vi "MicTest.vi"() -> ()   [LabVIEW 2024]
uses:
  ViolinSubs/PreferencesControl.ctl
  <vilib>/Analysis/5stat.llb/RMS (DBL).vi
  <extravilib>/ChannelInstances/Lossy Stream-a[.](wfm(dbl))/Read With Abort.vi
  <extravilib>/ChannelInstances/Lossy Stream-a[.](wfm(dbl))/EndpointRead.vi
  <extravilib>/ChannelInstances/Lossy Stream-a[.](wfm(dbl))/Instantiate.vi
  <extravilib>/ChannelInstances/Lossy Stream-a[.](wfm(dbl))/)Channel.vi
  <resource>/ChannelSupport/_ChannelSupport/WaitIfNeeded.vi
  <extravilib>/ChannelInstances/Lossy Stream-a[.](wfm(dbl)).lvlib
  <vilib>/Analysis/NI_AALPro.lvlib
panel:
  out "Hammer 2":waveform(dbl)(graph)={"t0"=timestamp(3623766685.135353 s since 1904-01-01), "dt"=2.0833333333333333e-05, "Y"=array[9600 elements]}
  out "Microphone 2":waveform(dbl)(graph)={"t0"=timestamp(3623766685.135353 s since 1904-01-01), "dt"=2.0833333333333333e-05, "Y"=array[9600 elements]}
  out "rms value 2":dbl format="%0.6f"
  out "peak 2":dbl
  out "peak":dbl
  out "rms value":dbl format="%0.6f"
  in  "device:":u16(ring)=1 items=["Built-in Microph", "Babyface Pro (71982712)"]
  out "Task":T1(ring)=enum."One Shot - waiting"
  out "Hammer":waveform(dbl)(graph)={"t0"=timestamp(3623766685.135353 s since 1904-01-01), "dt"=2.0833333333333333e-05, "Y"=array[9600 elements]}
  out "Microphone":waveform(dbl)(graph)={"t0"=timestamp(3623766685.135353 s since 1904-01-01), "dt"=2.0833333333333333e-05, "Y"=array[9600 elements]}
  in  "stop":bool
  in  "Settings":T2={"Name of test"="ScratchPad", "Date"=timestamp(3622387832 s since 1904-01-01), "Location"="Home", "Template"="ScratchPad", "Soundcard"="OCTA-CAPTURE", "resolution"=32, "Sampling rate"=48000, "Ch1 Gain "=20.0, "Ch2 Gain"=20.0, "Sample time (s)"=0.3, "Pre-trigger (s)"=0.001, "Hammer Threshold"=0.01, "Positions"=2, "Taps/Position"=2, "Set Names"="H,V", "Freq resolution"=1.0, "Hammer cutoff"=0.025, "Mic cutoff"=0.25, "Double bounce "=0.01, "Hammer Cal"=1.0, "dB Offset"=0.0, "Accel Cal"=1.0, "Vibrometer Cal"=20.0, "Mic Cal"=49.38, "Output"=2, "Voltage Cal"=13.8, "Vibrometer Port"="ASRL27::INSTR", "Range"=4, "High Pass"=2, "Bandwidth"=4, "X Range"=[{"Minimum"=200.0, "Maximum"=10000.0, "Increment"=10.0, "Minor Increment"=100.0, "Start"=200.0}, {"Minimum"=0.0, "Maximum"=0.05, "Increment"=0.025, "Minor Increment"=0.0025, "Start"=0.0}, {"Minimum"=0.0, "Maximum"=0.3, "Increment"=0.1, "Minor Increment"=0.01, "Start"=0.0}, {"Minimum"=200.0, "Maximum"=10000.0, "Increment"=10.0, "Minor Increment"=100.0, "Start"=1000.0}], "Y Range"=[{"Minimum"=-25.0, "Maximum"=0.0, "Increment"=5.0, "Minor Increment"=1.0, "Start"=-25.0}, {"Minimum"=-0.01, "Maximum"=0.1, "Increment"=0.02, "Minor Increment"=0.005, "Start"=0.0}, {"Minimum"=-0.1, "Maximum"=0.1, "Increment"=0.05, "Minor Increment"=0.01, "Start"=-0.1}, {"Minimum"=-35.0, "Maximum"=5.0, "Increment"=2.0, "Minor Increment"=0.5, "Start"=-34.0}], "dB Spread"=40.0, "Trigger"=0, "Ch_1"=1, "Ch_2"=2, "flip?"=FALSE, "60Hz"=FALSE, "Time offset"=0.0, "Piezo Cal"=1.0, "Default Notes"=""} {"Ch_2" min=1 step=1; "Ch_1" min=1 max=100 step=1; "Trigger" items=["Hammer (force)", "Self-tap", "Spacebar"]; "Bandwidth" items=["1 kHz"=1, "5 kHz"=5, "10 kHz"=10, "25 kHz"=25, "50 kHz"=50, "100 kHz"=100]; "High Pass" items=["Off", "13 Hz", "104 Hz"]; "Range" items=["10 mm/s"=1, "20 mm/s"=2, "50 mm/s"=5, "100 mm/s"=10, "200 mm/s"=20, "500 mm/s"=50, "1 m/s"=100, "2 m/s"=200]; "Output" items=["Accelerometer", "Speed (from acceleration)", "Microphone", "Vibrometer", "Piezo"]; "Voltage Cal" format="%#_13g"; "Ch2 Gain" format="%#_13g"; "Ch1 Gain" format="%#_13g"; "Double bounce" min=0.0; "Mic cutoff" min=0.0 format="%#_4g"; "Hammer cutoff" min=0.0 format="%#_4g"; "Freq resolution" min=0.0; "Pre-trigger (s)" format="%#_13g"; "Date" format="%<%H:%M\n%d/%m/%y>T"; "resolution" items=["16 bit"=16, "24 bit"=24, "32 bit"=32]; "Sampling rate" items=["22050 samp/s"=22050, "44100 samp/s"=44100, "48000 samp/s"=48000]}
  # "Babyface Pro (71982712)\n\nOCTACAPTURE\n\nBuilt-in Microph"
  # "Hz"
  # "dB"
  # "dB"
  # "sec"
  # "sec"
  # "mV/Pa"
  # "mV/m/s2"
  # "mV/mm/s"
  # "V/N"
  # "sec"
  # "sec"
  # "mV/N"
  # "a.u."
  # "a.u."
  # "sec"
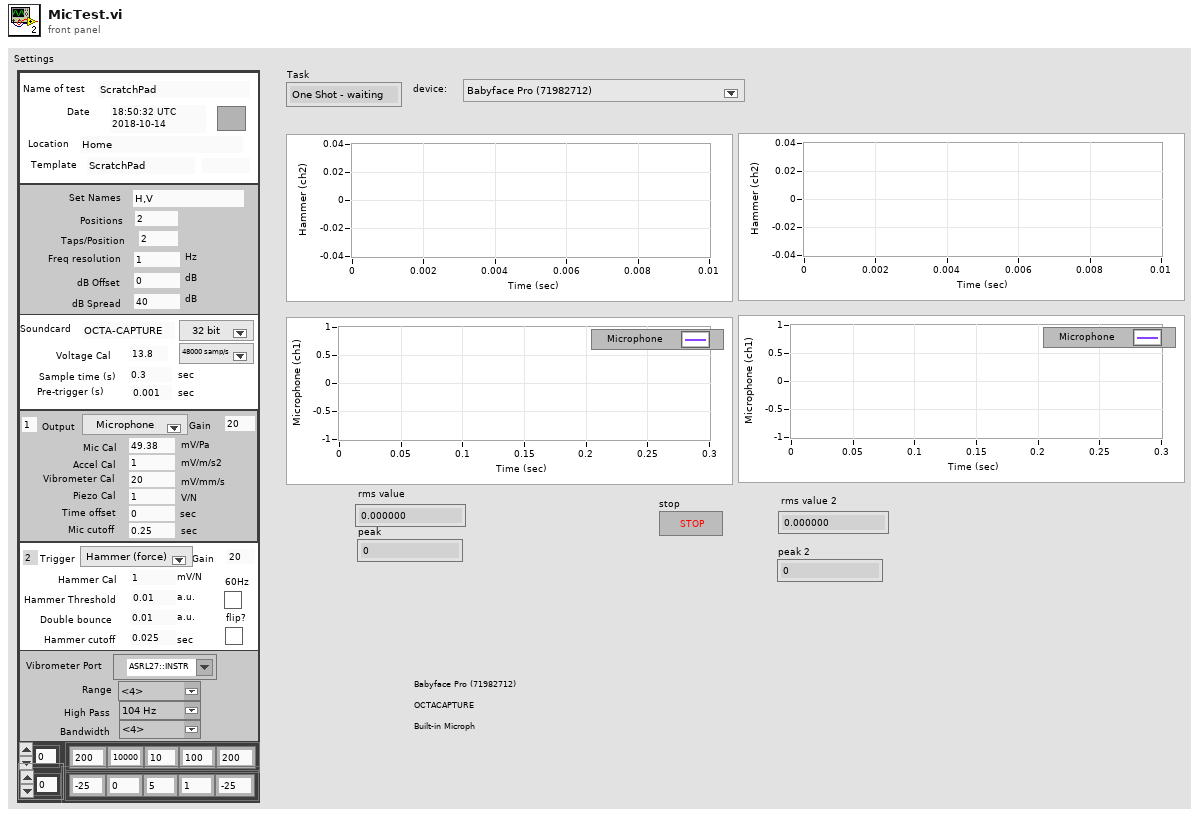
[diagram p1: front panel]
types:
  T1 = enum16{"Initialize", "Free run", "One Shot - waiting", "One Shot - triggered", "Wait", "Close"}
  T2 = typedef "PreferencesControl.ctl" = cluster{"Name of test":string, "Date":timestamp, "Location":string, "Template":string, "Soundcard":string, "resolution":u16, "Sampling rate":u16, "Ch1 Gain ":dbl, "Ch2 Gain":dbl, "Sample time (s)":dbl, "Pre-trigger (s)":dbl, "Hammer Threshold":dbl, "Positions":i16, "Taps/Position":i16, "Set Names":string, "Freq resolution":dbl, "Hammer cutoff":dbl, "Mic cutoff":dbl, "Double bounce ":dbl, "Hammer Cal":dbl, "dB Offset":dbl, "Accel Cal":dbl, "Vibrometer Cal":dbl, "Mic Cal":dbl, "Output":u16, "Voltage Cal":dbl, "Vibrometer Port":refnum<visa-resource-name>, "Range":u16, "High Pass":u16, "Bandwidth":u16, "X Range":cluster{"Minimum":dbl, "Maximum":dbl, "Increment":dbl, "Minor Increment":dbl, "Start":dbl}[], "Y Range":cluster{"Minimum":dbl, "Maximum":dbl, "Increment":dbl, "Minor Increment":dbl, "Start":dbl}[], "dB Spread":dbl, "Trigger":u16, "Ch_1":u8, "Ch_2":u8, "flip?":bool, "60Hz":bool, "Time offset":dbl, "Piezo Cal":dbl, "Default Notes":string}
  T3 = typedef "Sound Input Task ID.ctl" = u32
  T4 = cluster{"task ID":T3, "Num Pts":i32, "timeout":dbl, "FIFO":i32, "Double Bounce":dbl}
  T5 = typedef "Lossy Stream-a[.](wfm(dbl)).lvlib/)Channel.ctl" = refnum<queue>
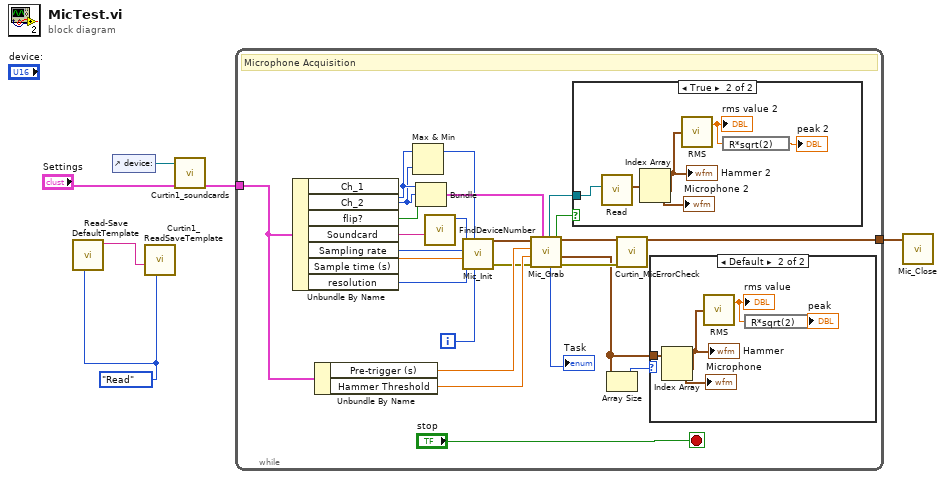
[diagram p0: block diagram]
diagram:
  w3 = enum16{"Save", "Read", "List"}."Read" ("Task")
  n1 = call "Read-Save DefaultTemplate.vi"("Task"=w3) -> ("Template Out"=w4:string)  [unwired: 9 in, 1 out]
  n2 = control-ref of="device:"() -> (w5:refnum<vi>)
  n3 = call "Curtin1_ReadSaveTemplate.vi"("Task"=w3, "Template"=w4) -> ()  [unwired: 6 in, 4 out]
  n4 = call "Curtin1_soundcards.vi"("Settings In"="Settings", "device:"=w5) -> ("Settings Out"=w2:T2)  [unwired: 8 in, 1 out]
  n5 = while {
    tunnel: [w30] -> w6
    tunnel: w2 -> [w18]
    i -> [w20]
    stop <- "stop" stop-if-true
    # "Microphone Acquisition"
    n6 = Unbundle By Name(w18) -> ("Ch_1"=w10:u8, "Ch_2"=w9:u8, "flip?"=w7:bool, "Soundcard"=w24:string, "Sampling rate"=w23:u16, "Sample time (s)"=w22:dbl, "resolution"=w21:u16)
    n7 = Unbundle By Name(w18) -> ("Pre-trigger (s)"=w29:dbl, "Hammer Threshold"=w28:dbl)
    n8 = Max & Min(x=w10, y=w9) -> (max(x,y)=w8:u8)  [unwired: 1 out]
    n9 = Bundle("Ch_1"=w10, "Ch_2"=w9, "flip?"=w7) -> (w11:cluster{"Ch_1":u8, "Ch_2":u8, "flip?":bool})  [unwired: 1 in]
    n10 = call "FindDeviceNumber.vi"("device"=w24) -> ("device"=w13:u16)  [unwired: 10 in]
    n11 = call "Mic_Init.vi"("itteration"=w20, "# channels"=w8, "resolution"=w21, "Sample time"=w22, "Sampling rate"=w23, "device"=w13) -> ("error out"=w26:errorcluster, "DAQ Prams"=w25:T4)  [unwired: 4 in]
    n12 = call "Mic_Grab.vi"("Ports"=w11, "error In"=w26, "Threshold"=w28, "Pre-trigger (s)"=w29, "DAQ Prams"=w25) -> ("error out"=w27:errorcluster, "latest data"=w15:waveform(dbl)[], "Full"=w12:bool, "DAQ Prams"=w30:T4, "Start Task"=→"Task":T1, "Tap"=w16:T5)  [unwired: 1 in]
    n13 = case shown="True" w12 {
      tunnel: w16 -> [_ w41]
      frame False {
      }
      frame True {
        n14 = call <extravilib>:"Read.vi"("channel"=w41) -> ("element"=w36:waveform(dbl)[])  [unwired: 5 in, 5 out]
        n15 = Index Array(array=w36) -> (element #1=w38:waveform(dbl), element #2=→"Microphone 2":waveform(dbl))  [unwired: 2 in]
        "Hammer 2" <- w38
        n16 = call-poly <vilib>:"RMS.vi"("X"=w38) -> ("rms value"=w39:dbl)  [unwired: 1 out]
        "rms value 2" <- w39
        n17 = expression code="R*sqrt(2)"(w39) -> (→"peak 2":dbl)
      }
    }
    n18 = Array Size(array=w15) -> (size(s)=w14:i32)
    n19 = call "Curtin_MicErrorCheck.vi"("error in (no error)"=w27) -> ()  [unwired: 11 in]
    n20 = case shown="Default" w14 {
      tunnel: w15 -> [_ w34]
      frame 0 {
      }
      frame Default {
        n21 = Index Array(array=w34) -> (element #1=w33:waveform(dbl), element #2=→"Microphone":waveform(dbl))  [unwired: 2 in]
        "Hammer" <- w33
        n22 = call-poly <vilib>:"RMS.vi"("X"=w33) -> ("rms value"=w32:dbl)  [unwired: 1 out]
        "rms value" <- w32
        n23 = expression code="R*sqrt(2)"(w32) -> (→"peak":dbl)
      }
    }
  }
  n24 = call "Mic_Close.vi"("DAQ Prams"=w6) -> ()  [unwired: 10 in, 1 out]
